vi "Run 01 Reset.vi"(11 "NXT/EV3 in":T1) -> (3 "NXT/EV3 out":T1)   [LabVIEW 2016]
uses:
  <vilib>/NXT/Subs/LVHSConnector.ctl
  <vilib>/NXT/LegoClasses/BrickReference/BrickReference.lvclass
  <vilib>/NXT/Block Support/NXT_OutputPort.ctl
  <vilib>/NXT/NXTIO Xnodes/NXTIONodeSubVIs/NXTMoveMotors.vi
  <vilib>/NXT/Dual Mode Library/Waits/Wait_Num.vi
  <vilib>/NXT/NXTIO Xnodes/NXTIONodeSubVIs/NXTStopMotors.vi
  <vilib>/NXT/NXTIO Xnodes/AddressXNode/NXTIOAddress.xnode
  <vilib>/NXT/NXTIO Xnodes/NXTIOXNode/NXTIO.xnode
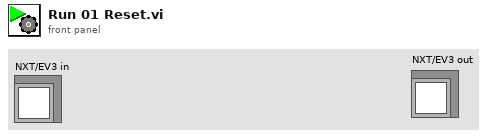
[diagram p1: front panel]
types:
  T1 = typedef "LVHSConnector.ctl" = refnum<class "BrickReference.lvclass">
  T2 = typedef "NXT_OutputPort.ctl" = u8
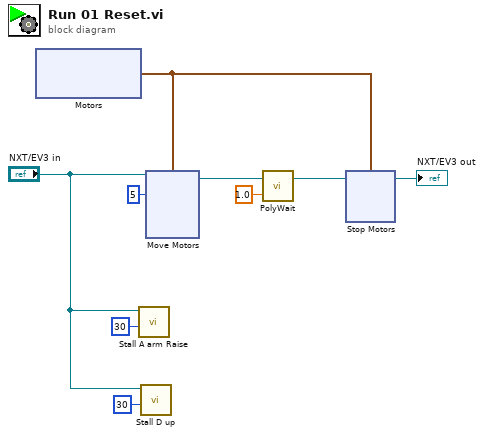
[diagram p0: block diagram]
diagram:
  w9 = i8 5 ("Power/Speed 1")
  n1 = xnode "Motors"() -> ("Motor"=w4:cluster{"Port":T2, "Port":T2})
  n2 = call "Stall A arm Raise.vi"("Power"=i8 30, "NXT/EV3"="NXT/EV3 in") -> ()  [unwired: 9 in, 1 out]
  n3 = call "Stall D up.vi"("Power"=i8 30, "NXT/EV3"="NXT/EV3 in") -> ()  [unwired: 9 in, 1 out]
  n4 = xnode "Move Motors"("Power/Speed 2"=w9, "Power/Speed 1"=w9, "Motors"=w4, "NXT/EV3"="NXT/EV3 in") -> ("NXT/EV3"=w8:T1)
  n5 = call-poly <vilib>:"PolyWait.vi"("Time (1 sec)"=sgl 1.0, "NXT/EV3"=w8) -> ("NXT/EV3"=w6:T1)  [unwired: 2 in]
  n6 = xnode "Stop Motors"("Motors"=w4, "NXT/EV3"=w6) -> ("NXT/EV3"=→"NXT/EV3 out":T1)
